vi "Configure Frequency.vi"(5 "Sweep time (ms)":dbl caption="Sweep time for zero span (ms)", 7 "Mode (Center/Span)":enum16{"Center/Span", "Start/Stop"}(ring), 8 "error in (no error)":errorcluster, 9 "Span/Stop Frequency [Hz]":dbl, 10 "Center/Start Frequency [Hz]":dbl, 11 "SA-FSW in":refnum<class "SA-FSW.lvclass">) -> (0 "error out":errorcluster, 3 "SA-FSW out":refnum<class "SA-FSW.lvclass">)   [LabVIEW 2020, in "SA-FSW.lvclass"]
uses:
  SA-FSW.lvclass
  C:/Sandbox/Git_Sandbox/WiSpry Test Framework source code (LV20)/WiSpry Test Framework/Instruments/Spectrum Analyzer/Spectrum Analyzer.lvclass
  C:/Sandbox/Git_Sandbox/WiSpry Test Framework source code (LV20)/WiSpry Test Framework/Instruments/Instrument.lvclass
  Spectrum Analyzer.lvclass/Spectrum Analyzer.ctl
  Instrument.lvclass/Instrument.ctl
  Instrument.lvclass
  Spectrum Analyzer.lvclass
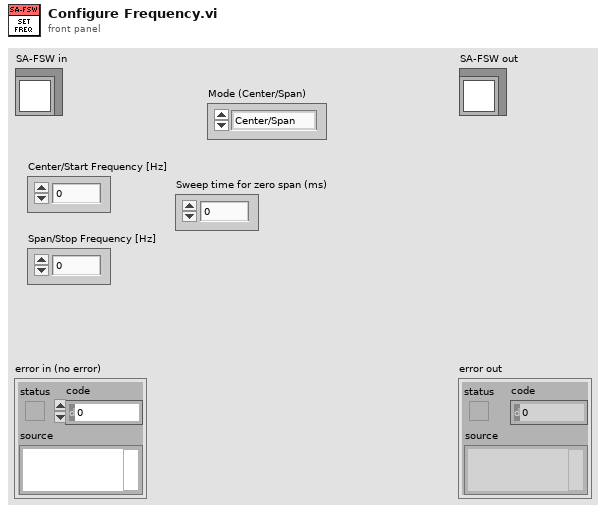
[diagram p1: front panel]
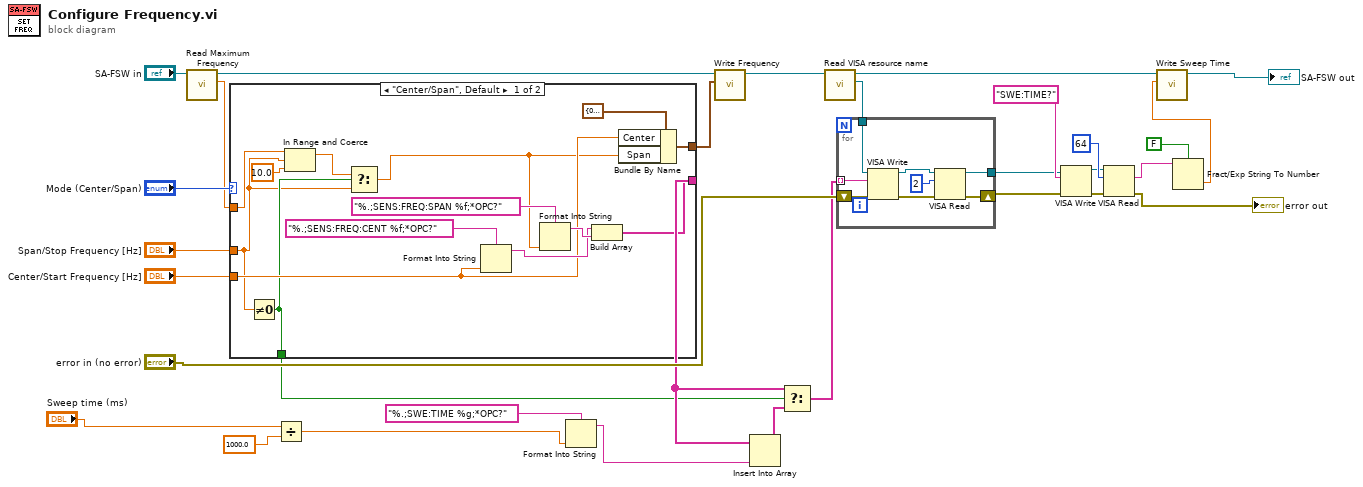
[diagram p0: block diagram]
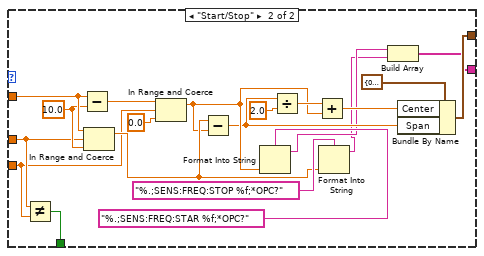
[diagram p2: hidden frame]
diagram:
  n1 = call "Read Maximum Frequency.vi"("Spectrum Analyzer in"="SA-FSW in") -> ("Maximum Frequency"=w27:dbl, "Spectrum Analyzer out"=w24:refnum<class "SA-FSW.lvclass">)  [unwired: 9 in]
  n2 = case shown="\"Center/Span\", Default" "Mode (Center/Span)" {
    tunnel: "Center/Start Frequency [Hz]" -> [w36 w47]
    tunnel: "Span/Stop Frequency [Hz]" -> [w32 w48]
    tunnel: w27 -> [w44 w62]
    tunnel: [w38 w49] -> w4
    tunnel: [w39 w52] -> w22
    tunnel: [w35 w46] -> w2
    frame "Center/Span", Default {
      n3 = Not Equal To 0?(x=w32) -> (x != 0?=w35:bool)
      n4 = In Range and Coerce(upper limit=w44, x=w32, lower limit=10.0) -> (coerced(x)=w34:dbl)  [unwired: 1 out]
      n5 = Select(t=w34, s=w35, f=w32) -> (s? t:f=w33:dbl)
      n6 = Format Into String(format string="%.;SENS:FREQ:CENT %f;*OPC?", w36) -> (resulting string=w37:string)  [unwired: 2 in, 1 out]
      n7 = Format Into String(format string="%.;SENS:FREQ:SPAN %f;*OPC?", w33) -> (resulting string=w41:string)  [unwired: 2 in, 1 out]
      n8 = Build Array(w37, w41) -> (w38:string[])
      n9 = Bundle By Name(cluster=cluster{"Center":dbl, "Span":dbl} {"Center"=0.0, "Span"=0.0} ("Frequency"), "Center"=w36, "Span"=w33) -> (w39:cluster{"Center":dbl, "Span":dbl})
    }
    frame "Start/Stop" {
      w61 = 10.0
      n10 = Not Equal?(x=w48, y=w47) -> (x != y?=w46:bool)
      n11 = Subtract(x=w62, y=w61) -> (x-y=w63:dbl)
      n12 = In Range and Coerce(upper limit=w62, x=w48, lower limit=w61) -> (coerced(x)=w59:dbl)  [unwired: 1 out]
      n13 = In Range and Coerce(upper limit=w63, x=w47, lower limit=0.0) -> (coerced(x)=w56:dbl)  [unwired: 1 out]
      n14 = Subtract(x=w59, y=w56) -> (x-y=w53:dbl)
      n15 = Format Into String(format string="%.;SENS:FREQ:STAR %f;*OPC?", w56) -> (resulting string=w51:string)  [unwired: 2 in, 1 out]
      n16 = Divide(x=w53, y=2.0) -> (x/y=w57:dbl)
      n17 = Add(x=w57, y=w56) -> (x+y=w54:dbl)
      n18 = Format Into String(format string="%.;SENS:FREQ:STOP %f;*OPC?", w59) -> (resulting string=w50:string)  [unwired: 2 in, 1 out]
      n19 = Build Array(w51, w50) -> (w49:string[])
      n20 = Bundle By Name(cluster=cluster{"Center":dbl, "Span":dbl} {"Center"=0.0, "Span"=0.0} ("Frequency"), "Center"=w54, "Span"=w53) -> (w52:cluster{"Center":dbl, "Span":dbl})
    }
  }
  n21 = Divide(x="Sweep time (ms)", y=1000.0) -> (x/y=w7:dbl)
  n22 = Format Into String(format string="%.;SWE:TIME %g;*OPC?", w7) -> (resulting string=w6:string)  [unwired: 2 in, 1 out]
  n23 = call "Write Frequency.vi"("Frequency"=w22, "Spectrum Analyzer in"=w24) -> ("Spectrum Analyzer out"=w23:refnum<class "SA-FSW.lvclass">)  [unwired: 9 in]
  n24 = Insert Into Array(array=w4, new element=w6) -> (w5:string[])  [unwired: 1 in]
  n25 = Select(t=w4, s=w2, f=w5) -> (s? t:f=w3:string[])
  n26 = call "Read VISA resource name.vi"("Instrument in"=w23) -> ("VISA resource name"=w26:refnum<visa-resource-name>, "Instrument out"=w12:refnum<class "SA-FSW.lvclass">)  [unwired: 9 in]
  n27 = for {
    tunnel: w26 -> [w73]
    shift-right: [w71] -> w16
    shift-left: "error in (no error)" -> [w72]
    tunnel: w3 -> [w67] mode=indexing
    tunnel: [w66] -> w15
    n28 = VISA Write(VISA resource name=w73, write buffer=w67, error in (no error)=w72) -> (VISA resource name out=w69:refnum<visa-resource-name>, error out=w70:errorcluster)  [unwired: 1 out]
    n29 = VISA Read(VISA resource name=w69, byte count=u32 2, error in (no error)=w70) -> (VISA resource name out=w66:refnum<visa-resource-name>, error out=w71:errorcluster)  [unwired: 2 out]
  }
  n30 = VISA Write(VISA resource name=w15, write buffer="SWE:TIME?", error in (no error)=w16) -> (VISA resource name out=w18:refnum<visa-resource-name>, error out=w13:errorcluster)  [unwired: 1 out]
  n31 = VISA Read(VISA resource name=w18, byte count=u32 64, error in (no error)=w13) -> (read buffer=w20:string, error out=→"error out":errorcluster)  [unwired: 2 out]
  n32 = Fract/Exp String To Number(use system decimal point (T)=FALSE, string=w20) -> (number=w10:dbl)  [unwired: 2 in, 1 out]
  n33 = call "Write Sweep Time.vi"("Sweep Time"=w10, "Spectrum Analyzer in"=w12) -> ("Spectrum Analyzer out"=→"SA-FSW out":refnum<class "SA-FSW.lvclass">)  [unwired: 9 in]
